vi "updateFrontEnd.vi"(8 "error in (no error)":errorcluster, 10 "Pane":refnum<vi>, 11 "ICSettingsViewer in":refnum<class "ICSettingsViewer.lvclass">) -> (0 "error out":errorcluster, 2 "Pane out":refnum<vi>, 3 "ICSettingsViewer out":refnum<class "ICSettingsViewer.lvclass">)   [LabVIEW 2011, in "Views.lvlib" / "Camera.lvlib" / "ICSettingsViewer.lvclass"]
uses:
  ICSettingsViewer.lvclass
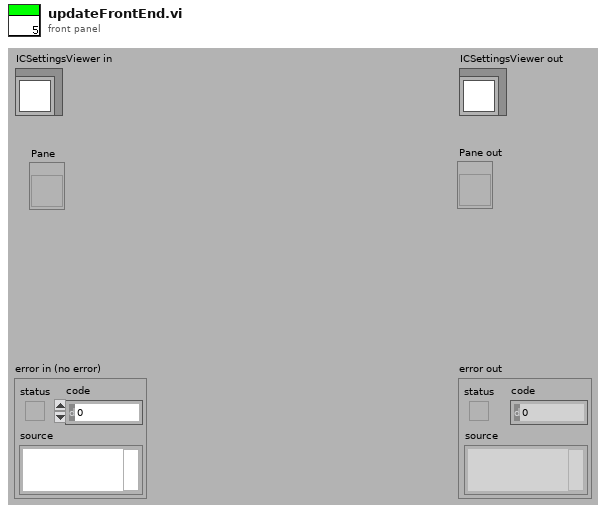
[diagram p1: front panel]
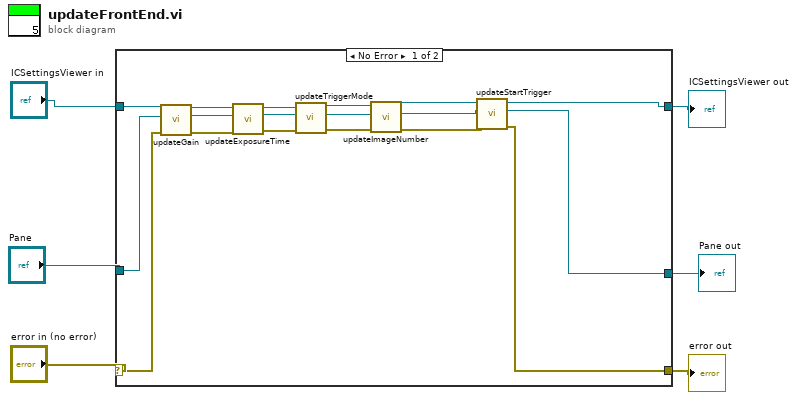
[diagram p0: block diagram]
diagram:
  n1 = case shown="No Error" "error in (no error)" {
    selector: "error in (no error)" -> [w23 w26]
    tunnel: [w10 w26] -> w5
    tunnel: [w7 w25] -> w3
    tunnel: "ICSettingsViewer in" -> [w24 w25]
    tunnel: "Pane" -> [w22 _]
    tunnel: [w8 _] -> w1
    frame No Error {
      n2 = call "updateGain.vi"("error in (no error)"=w23, "Pane"=w22, "ICSettingsViewer in"=w24) -> ("error out"=w19:errorcluster, "Pane out"=w20:refnum<vi>, "ICSettingsViewer out"=w21:refnum<class "ICSettingsViewer.lvclass">)  [unwired: 6 in]
      n3 = call "updateExposureTime.vi"("error in (no error)"=w19, "Pane"=w20, "ICSettingsViewer in"=w21) -> ("error out"=w18:errorcluster, "Pane out"=w16:refnum<vi>, "ICSettingsViewer out"=w17:refnum<class "ICSettingsViewer.lvclass">)  [unwired: 6 in]
      n4 = call "updateTriggerMode.vi"("error in (no error)"=w18, "Pane"=w16, "ICSettingsViewer in"=w17) -> ("error out"=w13:errorcluster, "Pane out"=w14:refnum<vi>, "ICSettingsViewer out"=w15:refnum<class "ICSettingsViewer.lvclass">)  [unwired: 6 in]
      n5 = call "updateImageNumber.vi"("error in (no error)"=w13, "Pane"=w14, "ICSettingsViewer in"=w15) -> ("error out"=w11:errorcluster, "Pane out"=w9:refnum<vi>, "ICSettingsViewer out"=w12:refnum<class "ICSettingsViewer.lvclass">)  [unwired: 6 in]
      n6 = call "updateStartTrigger.vi"("error in (no error)"=w11, "Pane"=w9, "ICSettingsViewer in"=w12) -> ("error out"=w10:errorcluster, "Pane out"=w8:refnum<vi>, "ICSettingsViewer out"=w7:refnum<class "ICSettingsViewer.lvclass">)  [unwired: 6 in]
    }
    frame Error {
    }
  }
  "error out" <- w5
  "ICSettingsViewer out" <- w3
  "Pane out" <- w1
